vi "myRIO_BRig_RT_dataMTrig_main__wWarmUp__v2__basic.vi"(0 "input_dataMTrig":u16[](array[numeric]), 4 "input_Audio_trig_L":bool) -> (14 "output_dataMTrig":u16[](array[numeric]), 18 "output_Audio_L":bool)   [LabVIEW 2014]
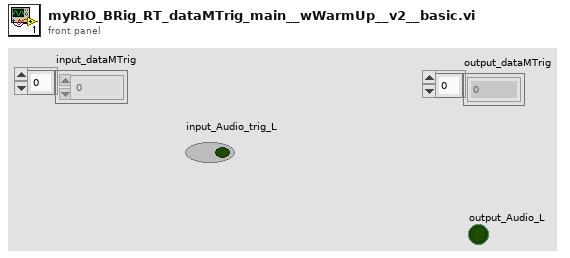
[diagram p1: front panel]
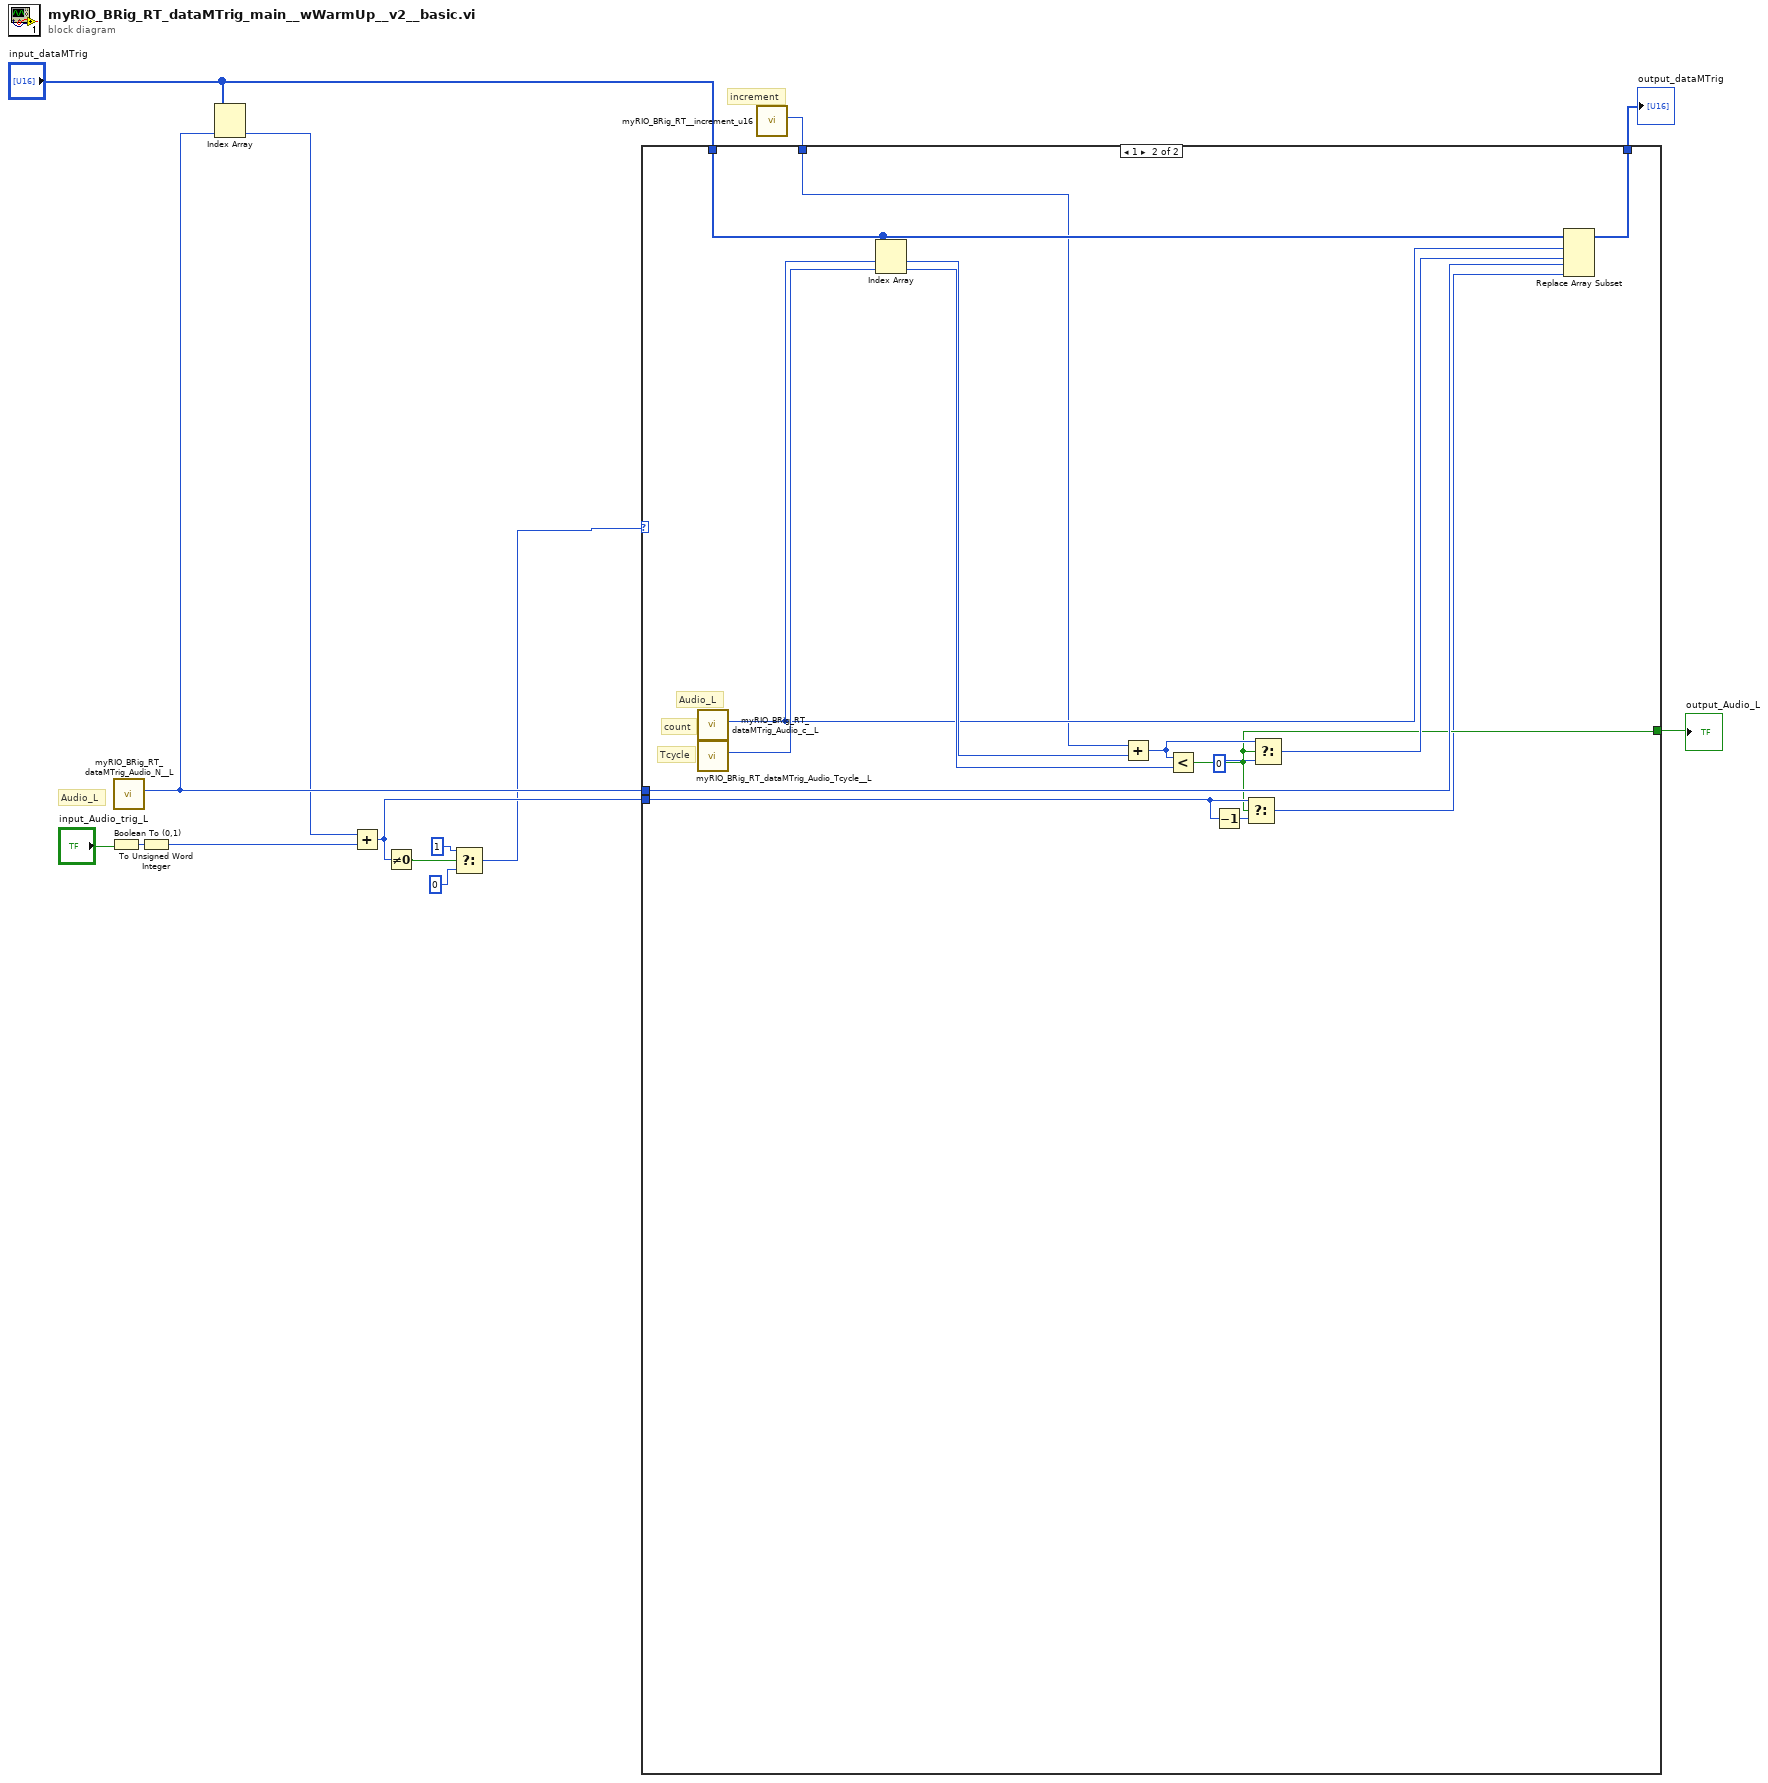
[diagram p0: block diagram]
diagram:
  # "increment"
  # "Audio_L"
  n1 = Boolean To (0,1)(Boolean="input_Audio_trig_L") -> (0, 1=w14:i16)
  n2 = call "myRIO_BRig_RT_dataMTrig_Audio_N__L.vi"() -> ("output_Audio_N__L"=w4:i32)  [unwired: 11 in]
  n3 = To Unsigned Word Integer(number=w14) -> (unsigned 16bit integer=w13:u16)
  n4 = Index Array(array="input_dataMTrig", index #2=w4) -> (element #2=w3:u16)  [unwired: 1 in, 1 out]
  n5 = Add(x=w3, y=w13) -> (x+y=w6:u16)
  n6 = Not Equal To 0?(x=w6) -> (x != 0?=w11:bool)
  n7 = Select(t=u8 1, s=w11, f=u8 0) -> (s? t:f=w2:u8)
  n8 = call "myRIO_BRig_RT__increment_u16.vi"() -> ("output_increment__u16"=w9:u16)  [unwired: 11 in]
  n9 = case shown="1" w2 {
    tunnel: "input_dataMTrig" -> [w15 w30]
    tunnel: w9 -> [_ w16]
    tunnel: [w15 w29] -> w8
    tunnel: w4 -> [_ w21]
    tunnel: w6 -> [_ w22]
    tunnel: [_ w18] -> w5
    frame 0, Default {
    }
    frame 1 {
      # "Audio_L"
      # "Tcycle"
      # "count"
      n10 = call "myRIO_BRig_RT_dataMTrig_Audio_c__L.vi"() -> ("output_Audio_c__L"=w20:i32)  [unwired: 11 in]
      n11 = call "myRIO_BRig_RT_dataMTrig_Audio_Tcycle__L.vi"() -> ("output_Audio_Tcycle__L"=w28:i32)  [unwired: 11 in]
      n12 = Index Array(array=w30, index #1=w20, index #2=w28) -> (element #1=w25:u16, element #2=w24:u16)
      n13 = Add(x=w16, y=w25) -> (x+y=w27:u16)
      n14 = Less?(x=w27, y=w24) -> (x < y?=w18:bool)
      n15 = Decrement(x=w22) -> (x-1=w23:u16)
      n16 = Select(t=w22, s=w18, f=w23) -> (s? t:f=w17:u16)
      n17 = Select(t=w27, s=w18, f=u16 0) -> (s? t:f=w19:u16)
      n18 = Replace Array Subset(array=w30, new element #1=w19, index #1=w20, new element #2=w17, index #2=w21) -> (w29:u16[])
    }
  }
  "output_dataMTrig" <- w8
  "output_Audio_L" <- w5
